vi "finishPrepareKeeperPassPlay.vi"(6 "Game":refnum<class "Game.lvclass">, 8 "error in (no error)":errorcluster, 9 "command_interpreted":T1, 11 "PrepareKeeperPassPlay in":refnum<class "PrepareKeeperPassPlay.lvclass">) -> (0 "error out":errorcluster, 2 "finished ?":bool, 3 "PrepareKeeperPassPlay out":refnum<class "PrepareKeeperPassPlay.lvclass">)   [LabVIEW 2020, in "PrepareKeeperPassPlay.lvclass"]
uses:
  PrepareKeeperPassPlay.lvclass
  Referee_class/command_interpreted.ctl
  Game_class/Game.lvclass
  Utilities_class/Utilities.lvclass
  Game_class/Game.lvclass/Game.ctl
  Team_class/Team.lvclass/Team.ctl
  Events_class/Events.lvclass/Events.ctl
  Game_class/Read BallRef.vi
  Game_class/Read KeeperTeam.vi
  Game_class/Read EventsRef.vi
  Events_class/Read touch.vi
  Events_class/Read id_touch.vi
  Team_class/Read RobotRef.vi
  Ally_class/Ally.lvclass
  Ball_class/Ball.lvclass
  Events_class/Events.lvclass
  Robot_class/Robot.lvclass
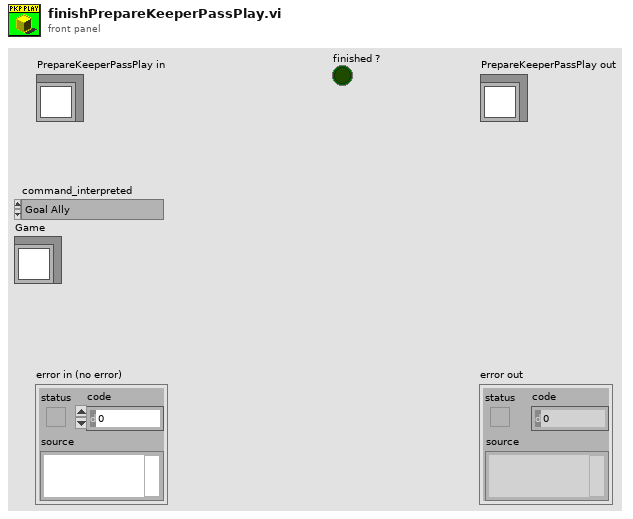
[diagram p1: front panel]
types:
  T1 = typedef "command_interpreted.ctl" = enum16{"Goal Ally", "Goal Enemy", "Ball Placement Enemy", "Ball Placement Ally", "Normal Half Time", "Extra Time  Break", "Extra Half Time", "None", "Post Game", "PKA Normal Start", "Prepare Kickoff Ally", "PKE Normal Start", "Prepare Kickoff Enemy", "Force Start", "Halt", "Timeout", "Prepare Penalty Ally", "Prepare Penalty Enemy", "PPA NormalStart", "PPE Normal Start", "Indirect Free Ally", "Direct Free Enemy", "Direct Free Ally", "Indirect Free Enemy", "Stop"}
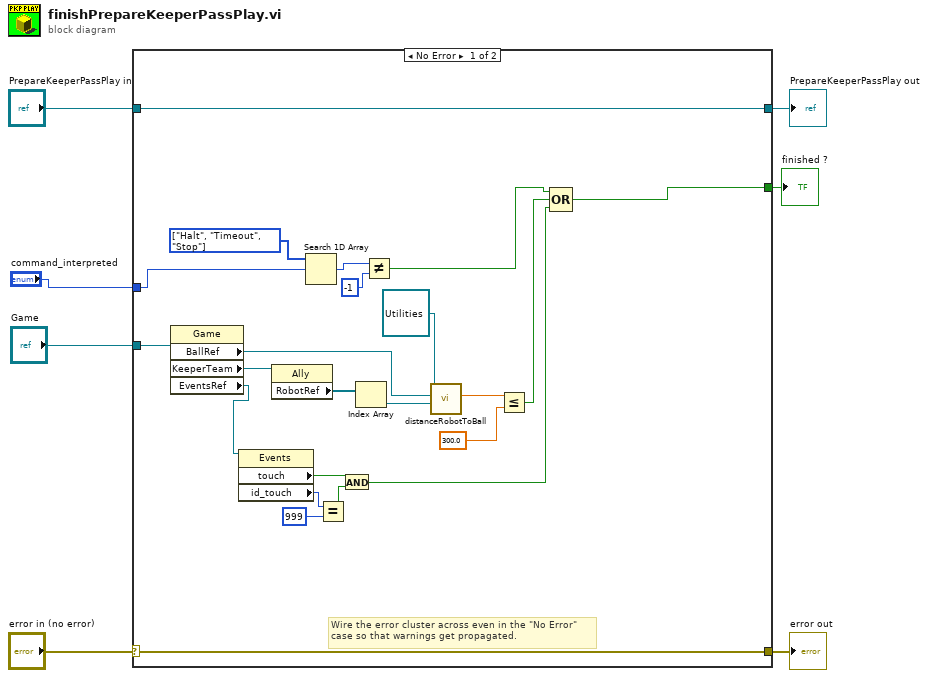
[diagram p0: block diagram]
diagram:
  n1 = case shown="No Error" "error in (no error)" {
    selector: "error in (no error)" -> [w29 w32]
    tunnel: [w29 w32] -> w6
    tunnel: [w30 w31] -> w4
    tunnel: "PrepareKeeperPassPlay in" -> [w30 w31]
    tunnel: "command_interpreted" -> [w27 _]
    tunnel: [w23 _] -> w2
    tunnel: "Game" -> [w22 _]
    frame No Error {
      w28 = T1[] [enum."Halt", enum."Timeout", enum."Stop"] items=["Goal Ally", "Goal Enemy", "Ball Placement Enemy", "Ball Placement Ally", "Normal Half Time", "Extra Time  Break", "Extra Half Time", "None", "Post Game", "PKA Normal Start", "Prepare Kickoff Ally", "PKE Normal Start", "Prepare Kickoff Enemy", "Force Start", "Halt", "Timeout", "Prepare Penalty Ally", "Prepare Penalty Enemy", "PPA NormalStart", "PPE Normal Start", "Indirect Free Ally", "Direct Free Enemy", "Direct Free Ally", "Indirect Free Enemy", "Stop"] ("Array")
      # "Wire the error cluster across even in the \"No Error\"\ncase so that warnings get propagated."
      n2 = property class="Game"(reference=w22) -> ("BallRef"=w18:refnum<class "Ball.lvclass">, "KeeperTeam"=w21:refnum<class "Ally.lvclass">, "EventsRef"=w13:refnum<class "Events.lvclass">)  [unwired: 1 in, 2 out]
      n3 = property class="Events"(reference=w13) -> ("touch"=w12:bool, "id_touch"=w11:i32)  [unwired: 1 in, 2 out]
      n4 = property class="Ally"(reference=w21) -> ("RobotRef"=w20:refnum<class "Robot.lvclass">[])  [unwired: 1 in, 2 out]
      n5 = Search 1D Array(1D array=w28, element=w27) -> (index of element=w26:i32)  [unwired: 1 in]
      n6 = Equal?(x=w11, y=999) -> (x = y?=w9:bool)
      n7 = And(x=w12, y=w9) -> (x .and. y?=w8:bool)
      n8 = Index Array(array=w20) -> (element=w19:refnum<class "Robot.lvclass">)  [unwired: 1 in]
      n9 = Not Equal?(x=w26, y=-1) -> (x != y?=w24:bool)
      n10 = call "distanceRobotToBall.vi"("Robot"=w19, "Ball"=w18, "Utilities in"=refnum<class "Utilities.lvclass"> refnum) -> ("Distance Robot To Ball"=w17:dbl)  [unwired: 6 in, 2 out]
      n11 = Less Or Equal?(x=w17, y=300.0) -> (x <= y?=w15:bool)
      n12 = Compound Arithmetic op=OR(w24, w15, w8) -> (w23:bool)
    }
    frame Error {
    }
  }
  "error out" <- w6
  "PrepareKeeperPassPlay out" <- w4
  "finished ?" <- w2
